vi "VIMain.vi"   [LabVIEW 2014]
doc: "This VI will be executed when the compiled executable is called."
uses:
  stdin.vi
  stdout.vi
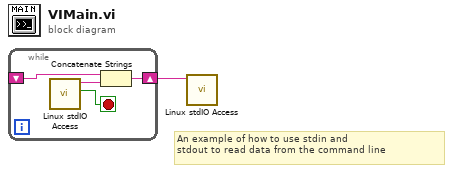
[diagram p0: block diagram]
diagram:
  # "An example of how to use stdin and\nstdout to read data from the command line"
  n1 = while {
    shift-right: [w4] -> w1
    shift-left: _ -> [w5]
    stop <- w2 stop-if-true
    n2 = call-poly "Linux stdIO Access.vi"() -> ("eof?"=w2:bool, "data"=w3:string)  [unwired: 4 in, 2 out]
    n3 = Concatenate Strings(w5, w3) -> (w4:string)
  }
  n4 = call-poly "Linux stdIO Access.vi"("data"=w1) -> ()  [unwired: 5 in, 2 out]
